vi "ClearCluster.vi"(8 "error in (no error)":errorcluster, 11 "GSstatus in":refnum<class "GSstatus.lvclass">) -> (0 "error out":errorcluster, 3 "GSstatus out":refnum<class "GSstatus.lvclass">)   [LabVIEW 2018, in "GSstatus.lvclass"]
uses:
  GSstatus.lvclass
  GSstatus.lvclass/GSstatus.ctl
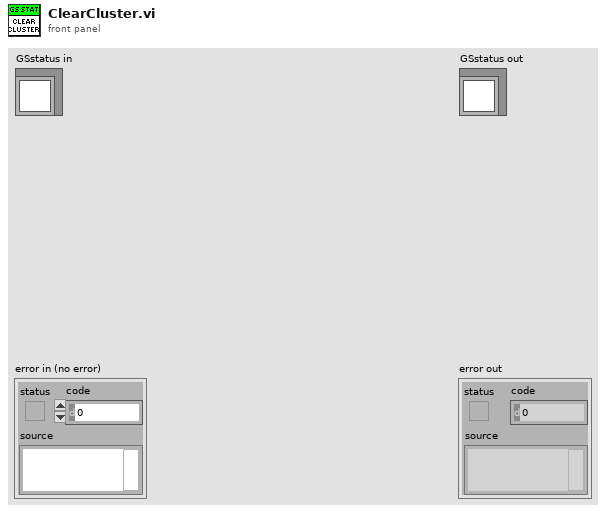
[diagram p1: front panel]
types:
  T1 = cluster{"FocusPhot":dbl, "FocusPolar":dbl, "FocusEffic":dbl, "FocusInstrum":dbl, "ICS":bool, "AG":bool, "BROKER":string, "timestamp":string, "FocusPos":dbl, "MirrorPos":dbl}
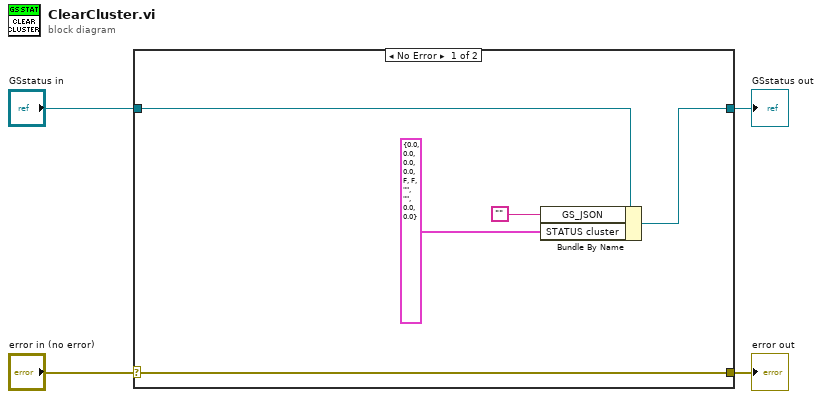
[diagram p0: block diagram]
diagram:
  n1 = case shown="No Error" "error in (no error)" {
    selector: "error in (no error)" -> [w9 w11]
    tunnel: [w9 w11] -> w3
    tunnel: [w7 w10] -> w1
    tunnel: "GSstatus in" -> [w8 w10]
    frame No Error {
      n2 = Bundle By Name(cluster=w8, "GS_JSON"="", "STATUS cluster"=T1 {"FocusPhot"=0.0, "FocusPolar"=0.0, "FocusEffic"=0.0, "FocusInstrum"=0.0, "ICS"=FALSE, "AG"=FALSE, "BROKER"="", "timestamp"="", "FocusPos"=0.0, "MirrorPos"=0.0}) -> (w7:refnum<class "GSstatus.lvclass">)
    }
    frame Error {
    }
  }
  "error out" <- w3
  "GSstatus out" <- w1
